vi "Create Test Configuration.vi"() -> (0 "error out":errorcluster, 1 "Names":string[](array[string]), 2 "Line Array":T1[](array[typedef]), 3 "module":refnum<class "dds configuration.lvclass">, 4 "Channels":refnum<class "TBM channel.lvclass">[](array[class]), 5 "instance identifier":string)   [LabVIEW 2020, in "dds tests.lvlib"]
doc: "This VI creates the test configuration used in testing. BY default just creates one line with every datatype"
uses:
  dds tests.lvlib
  module/configuration/dds configuration.lvclass
  C:/Program Files (x86)/National Instruments/LabVIEW 2020/vi.lib/NI/Configuration Framework/serializable configuration/NISE_CEF_serializable configuration.lvclass
  module/configuration/Line.ctl
  <vilib>/NI/Tag Bus Module Framework/channel/TBM channel.lvclass
  <vilib>/RTI DDS Toolkit/Types/RTI DDS Advanced Reader Configuration.ctl
  <vilib>/NI/Tag Bus Module Framework/channel/channel classification.ctl
  <vilib>/NI/Configuration Framework/serializable configuration/NISE_CEF_serializable configuration.lvclass
  <vilib>/RTI DDS Toolkit/Library/LVDDS_library.lvlib
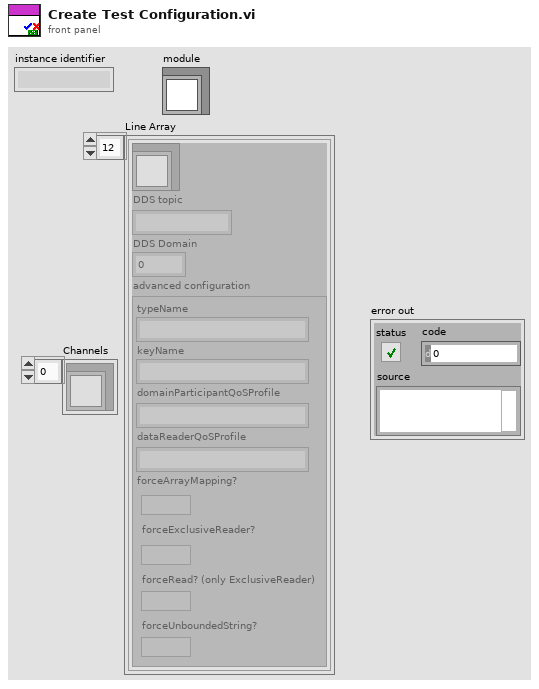
[diagram p1: front panel]
types:
  T1 = typedef "DDS configuration.lvclass/Line.ctl" = cluster{"channel":refnum<class "TBM channel.lvclass">, "DDS topic":string, "DDS Domain":u32, "advanced configuration":T2}
  T2 = typedef "LVDDS_library.lvlib/RTI DDS Advanced Reader Configuration.ctl" = cluster{"typeName":string, "keyName":string, "domainParticipantQoSProfile":string, "dataReaderQoSProfile":string, "forceArrayMapping?":bool, "forceExclusiveReader?":bool, "forceRead? (only ExclusiveReader)":bool, "forceUnboundedString?":bool}
  T3 = typedef "TBM channel.lvclass/channel classification.ctl" = enum16{"input data", "output data", "processing parameter", "processing result"}
  T4 = typedef "tag bus.lvlib/tag descriptor.lvclass/Data Type.ctl" = enum16{"Double", "Single", "I64", "I32", "I16", "I8", "U64", "U32", "U16", "U8", "Boolean", "String", "Array of Double", "Array of Single", "Array of I64", "Array of I32", "Array of I16", "Array of I8", "Array of U64", "Array of U32", "Array of U16", "Array of U8", "Array of Boolean", "Array of String"}
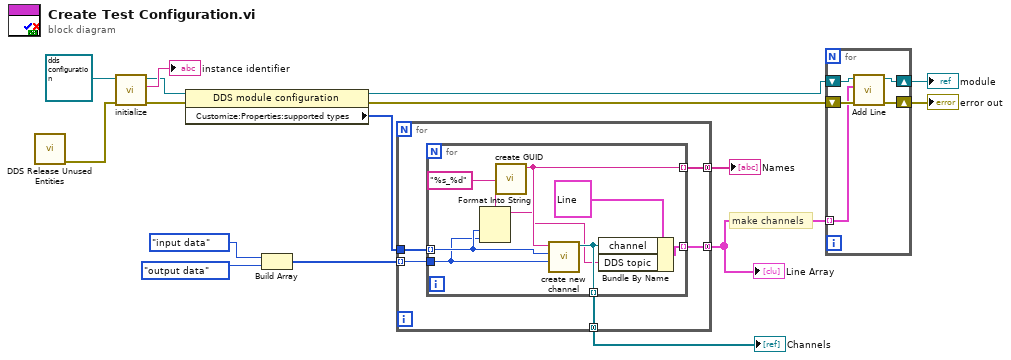
[diagram p0: block diagram]
diagram:
  # "make channels"
  n1 = call <vilib>:"DDS Release Unused Entities.vi"() -> ("error out"=w2:errorcluster)  [unwired: 10 in, 1 out]
  n2 = call <vilib>:"initialize.vi"("error in"=w2, "configuration in"=refnum<class "dds configuration.lvclass"> refnum ("tag bus configurable plugin module configuration")) -> ("error out"=w14:errorcluster, "identifier"=→"instance identifier":string, "configuration out"=w11:refnum<class "dds configuration.lvclass">)  [unwired: 7 in]
  n3 = property class="DDS module configuration"(reference=w11, error in=w14) -> (reference out=w7:refnum<class "dds configuration.lvclass">, error out=w13:errorcluster, "Customize:Properties:supported types"=w8:T4[])
  n4 = Build Array(channel_classification."input data" ("channel classification"), channel_classification."output data" ("channel classification")) -> (w6:T3[])
  n5 = for {
    tunnel: w6 -> [w21] mode=indexing
    tunnel: [w19] -> w1 mode=concatenating
    tunnel: w8 -> [w20]
    tunnel: [w18] -> w12 mode=concatenating
    tunnel: [w17] -> w3 mode=concatenating
    n6 = for {
      tunnel: w21 -> [w22]
      tunnel: [w27] -> w19 mode=indexing
      tunnel: w20 -> [w25] mode=indexing
      tunnel: [w29] -> w18 mode=indexing
      tunnel: [w26] -> w17 mode=indexing
      n7 = Format Into String(format string="%s_%d", w25, w22) -> (resulting string=w23:string)  [unwired: 2 in, 1 out]
      n8 = call <vilib>:"create GUID.vi"() -> ("uuid"=w29:string)  [unwired: 10 in, 1 out]
      n9 = call <vilib>:"create new channel.vi"("channel classification"=w22, "data type"=w25, "channel name"=w29) -> ("channel"=w26:refnum<class "TBM channel.lvclass">)  [unwired: 8 in]
      n10 = Bundle By Name(cluster=T1 {"channel"=refnum, "DDS topic"="", "DDS Domain"=0, "advanced configuration"={"typeName"="", "keyName"="", "domainParticipantQoSProfile"="", "dataReaderQoSProfile"="", "forceArrayMapping?"=FALSE, "forceExclusiveReader?"=FALSE, "forceRead? (only ExclusiveReader)"=FALSE, "forceUnboundedString?"=FALSE}} ("Line"), "channel"=w26, "DDS topic"=w23) -> (w27:T1)
    }
  }
  "Names" <- w12
  "Line Array" <- w1
  "Channels" <- w3
  n11 = for {
    tunnel: w1 -> [w30] mode=indexing
    shift-right: [w33] -> w10
    shift-left: w7 -> [w34]
    shift-right: [w31] -> w16
    shift-left: w13 -> [w32]
    n12 = call "Add Line.vi"("error in"=w32, "Line"=w30, "dds configuration in"=w34) -> ("error out"=w31:errorcluster, "dds configuration out"=w33:refnum<class "dds configuration.lvclass">)  [unwired: 7 in]
  }
  "error out" <- w16
  "module" <- w10
